vi "todos los modulos.vi"() -> ()   [LabVIEW 2010]
uses:
  <vilib>/sound2/lvsound2.llb/Sound Data Format.ctl
  <vilib>/addons/PixeLINK/Low Level Functions/CAMERA_FEATURES.llb/TDPU-CameraFeatures-PixelFormat.ctl
  <vilib>/sound2/lvsound2.llb/Sound Output Task ID.ctl
  <vilib>/vision/Image Controls.llb/IMAQ Image.ctl
panel:
  in  "Tab Control":enum32{"DAQ", "Sound", "Camara"}(tab)
  out "Waveform DAQ":waveform(dbl)(graph)
  in  "Calibracion DAQ":T1
  in  "DAQ Controls":T2={"Minimum Value"=-10.0, "Maximum Value"=10.0, "Physical Channel"="Dev1/ao0", "DAQ Fs (S/s)"=10000.0} {"Minimum Value" min=-10.0 max=0.0; "Maximum Value" min=0.0 max=10.0}
  in  "tiempo (ms)":dbl
  in  "DAQ?":bool
  in  "Sound Controls":T4={"device ID"=0, "sound format"={"sample rate (S/s)"=44000.0, "number of channels"=2, "bits per sample"=16}, "time (ms)"=200.0}
  in  "Sound?":bool
  in  "Frecuencia":dbl
  out "Waveform Sound":waveform(dbl)(graph)
  in  "Selector":u16(ring) items=["776002034"]
  in  "Streeam?":bool
  in  "Camera Parameters":T6 {"Pixel Format" items=["PIXEL_FORMAT_MONO8", "PIXEL_FORMAT_MONO16", "PIXEL_FORMAT_YUV422", "PIXEL_FORMAT_BAYER8_GRBG", "PIXEL_FORMAT_BAYER16_GRBG", "PIXEL_FORMAT_RGB24", "PIXEL_FORMAT_RGB48", "PIXEL_FORMAT_BAYER8_RGGB", "PIXEL_FORMAT_BAYER8_GBRG ", "PIXEL_FORMAT_BAYER8_BGGR ", "PIXEL_FORMAT_BAYER16_RGGB ", "PIXEL_FORMAT_BAYER16_GBRG", "PIXEL_FORMAT_BAYER16_BGGR", "PIXEL_FORMAT_RGB32"]}
  out "Camara Funciona?":bool
  out "Contraste":dbl
  out "Image":T7(plugin-control)
  in  "stop":bool
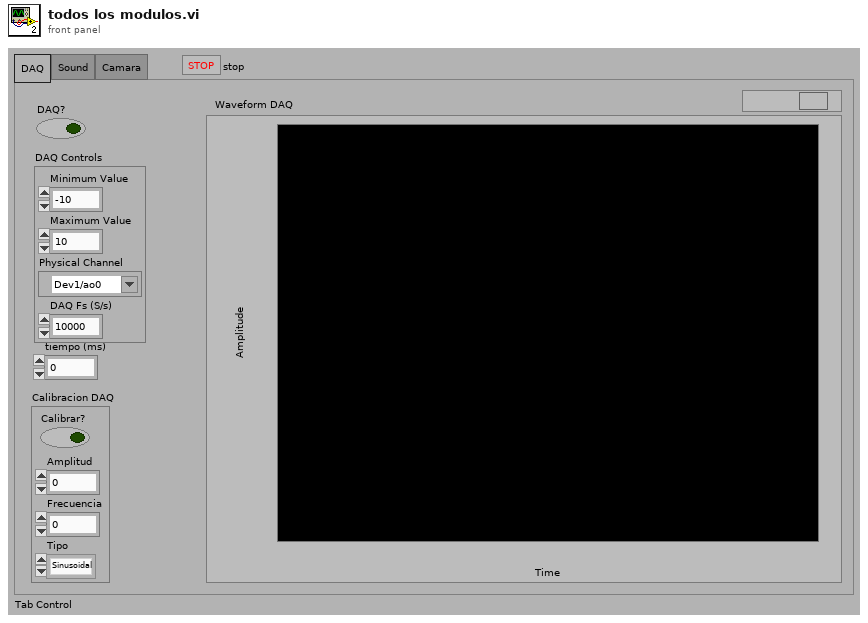
[diagram p1: front panel]
types:
  T1 = cluster{"Calibrar?":bool, "Amplitud":dbl, "Frecuencia":dbl, "Tipo":enum16{"Sinusoidal", "Triangular", "Cuadrada"}}
  T2 = cluster{"Minimum Value":dbl, "Maximum Value":dbl, "Physical Channel":tag, "DAQ Fs (S/s)":dbl}
  T3 = typedef "Sound Data Format.ctl" = cluster{"sample rate (S/s)":dbl, "number of channels":i32, "bits per sample":i32}
  T4 = cluster{"device ID":u32, "sound format":T3, "time (ms)":dbl}
  T5 = typedef "TDPU-CameraFeatures-PixelFormat.ctl" = u16
  T6 = cluster{"Exposure Time (ms)":u32, "Gain (dB)":dbl, "Saturation (%)":dbl, "Brightness (%)":dbl, "Color Temperature":dbl, "ROI":cluster{"Top":i32, "Left":i32, "Width":i32, "Height":i32}, "White Balance Gain (dB)":cluster{"Red":dbl, "Green":dbl, "Blue":dbl}, "Gamma":dbl, "Pixel Format":T5}
  T7 = typedef "IMAQ Image.ctl" = refnum<image>
  T8 = cluster{"hCamera":u32, "Error":errorcluster, "uSerialNumber OUT":u32}
  T9 = typedef "Sound Output Task ID.ctl" = u32
  T10 = cluster{"task ID":T9, "error":errorcluster, "sound format":T3}
  T11 = cluster{"DAQ Fs (S/s)":dbl, "task":refnum<k21>, "error":errorcluster, "Min Value":dbl, "Max Value":dbl}
  T12 = cluster{"DAQ Limits":cluster{"max":dbl, "min":dbl}, "Control Limits":cluster{"max":dbl, "min":dbl}}
  T13 = cluster{"hCamera":u32, "Error":errorcluster, "uSerialNumber":u32}
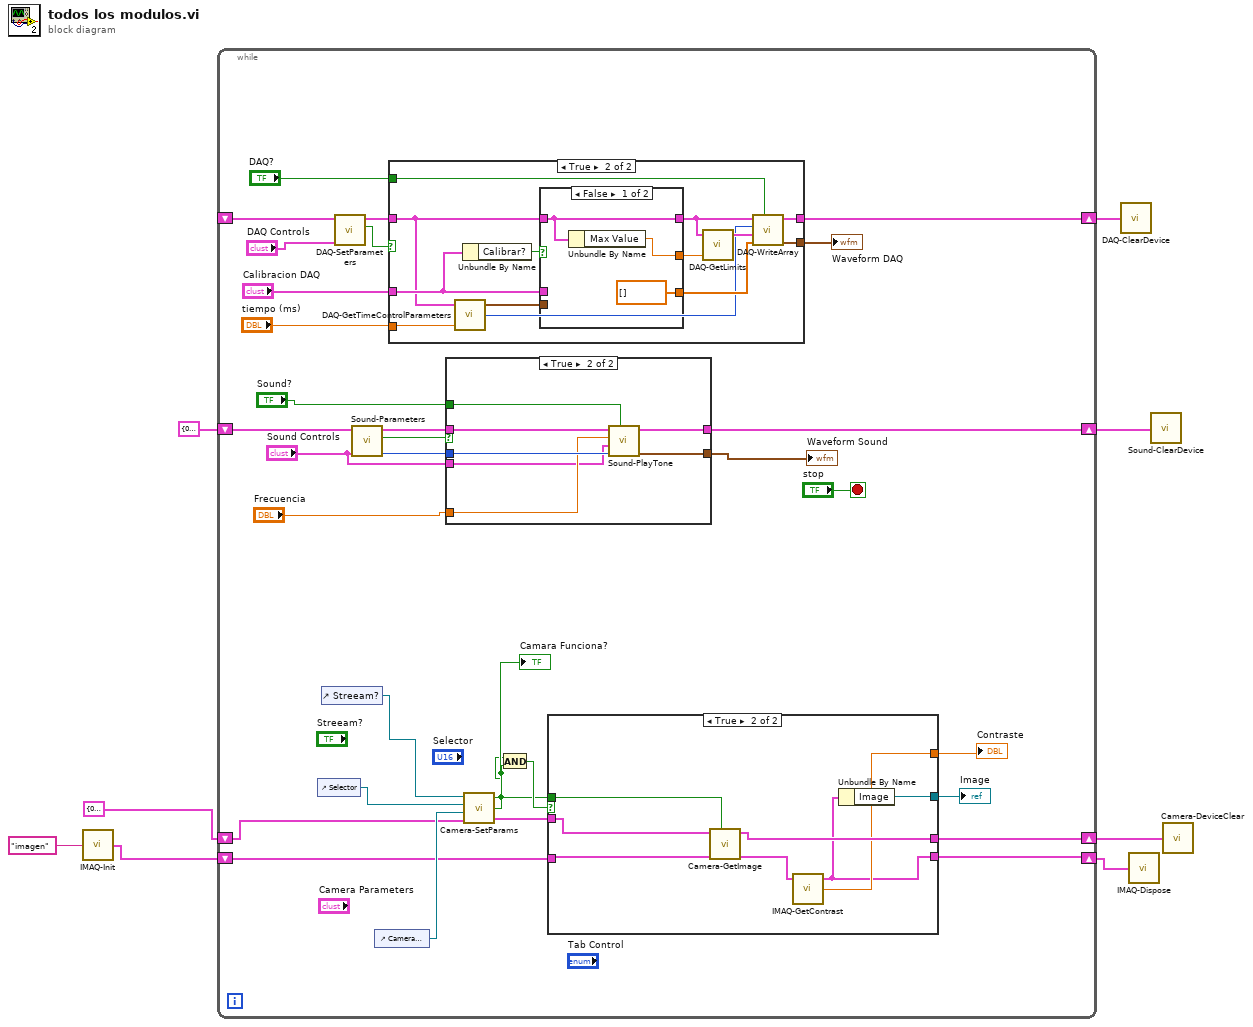
[diagram p0: block diagram]
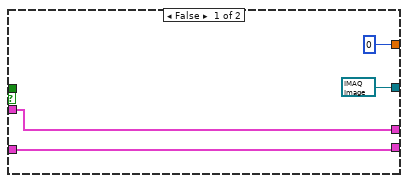
[diagram p2: hidden frame]
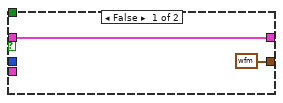
[diagram p3: hidden frame]
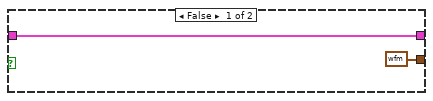
[diagram p4: hidden frame]
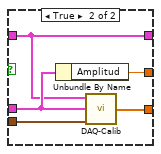
[diagram p5: hidden frame]
diagram:
  n1 = call "IMAQ-Init.vi"("Image Name"="imagen") -> ("Image Device IN"=w4:cluster{"Image":T7, "errorImage":errorcluster})
  n2 = while {
    shift-right: [w32] -> w6
    shift-left: _ -> [w33]
    shift-right: [w28] -> w7
    shift-left: T10 {"task ID"=0, "error"={"status"=TRUE, "code"=0, "source"=""}, "sound format"={"sample rate (S/s)"=0.0, "number of channels"=0, "bits per sample"=0}} ("Sound Device OUT") -> [w27]
    shift-right: [w13] -> w1
    shift-left: w4 -> [w17]
    shift-right: [w16] -> w2
    shift-left: T8 {"hCamera"=0, "Error"={"status"=FALSE, "code"=0, "source"=""}, "uSerialNumber OUT"=0} ("Camera Device  IN") -> [w15]
    stop <- "stop" stop-if-true
    n3 = control-ref of="Selector"() -> (w21:refnum<vi>)
    n4 = control-ref of="Streeam?"() -> (w19:refnum<vi>)
    n5 = call "DAQ-SetParameters.vi"("DAQ Controls"="DAQ Controls", "DAQ Device IN"=w33) -> ("En Funcionamiento?"=w26:bool, "DAQ Device OUT"=w38:T11)  [unwired: 4 in]
    n6 = call "Sound-Parameters.vi"("Sound Controls"="Sound Controls", "Sound Device IN"=w27) -> ("#samples"=w29:u32, "En funcionamiento?"=w25:bool, "Sound Device OUT"=w30:T10)  [unwired: 3 in]
    n7 = control-ref of="Camera Parameters"() -> (w20:refnum<vi>)
    n8 = case shown="True" w26 {
      tunnel: "DAQ?" -> [_ w74]
      tunnel: w38 -> [w63 w65]
      tunnel: [waveform(dbl) {"t0"=timestamp(0 s since 1904-01-01), "dt"=1.0, "Y"=[]} ("Waveform Graph") w71] -> w37
      tunnel: "Calibracion DAQ" -> [_ w67]
      tunnel: "tiempo (ms)" -> [_ w69]
      tunnel: [w63 w68] -> w32
      frame False {
      }
      frame True {
        n9 = call "DAQ-GetTimeControlParameters.vi"("tiempo (ms)"=w69, "DAQ Device IN"=w65) -> ("#samples"=w72:u32, "Time Control Parameters"=w73:cluster{"# samples":u32, "tiempos (ms)":dbl})  [unwired: 2 in]
        n10 = Unbundle By Name(w67) -> ("Calibrar?"=w66:bool)
        n11 = case shown="False" w66 {
          tunnel: [dbl[] [] ("Calibration OUT") w84] -> w76
          tunnel: w73 -> [_ w83]
          tunnel: w65 -> [w77 w80]
          tunnel: w67 -> [_ w82]
          tunnel: [w78 w81] -> w70
          tunnel: [w77 w80] -> w64
          frame False {
            n12 = Unbundle By Name(w77) -> ("Max Value"=w78:dbl)
          }
          frame True {
            n13 = Unbundle By Name(w82) -> ("Amplitud"=w81:dbl)
            n14 = call "DAQ-Calib.vi"("Time Control Parameters"=w83, "Calibracion DAQ"=w82, "DAQ Device IN"=w80) -> ("Calibration OUT"=w84:dbl[])  [unwired: 1 in]
          }
        }
        n15 = call "DAQ-GetLimits.vi"("Amplitud"=w70, "DAQ Device IN"=w64) -> ("Limites"=w75:T12)  [unwired: 3 in]
        n16 = call "DAQ-WriteArray.vi"("DAQ?"=w74, "Control Array"=w76, "Limites"=w75, "#samples"=w72, "DAQ Device IN"=w64) -> ("Waveform Graph"=w71:waveform(dbl), "DAQ Device OUT"=w68:T11)  [unwired: 2 in]
      }
    }
    "Waveform DAQ" <- w37
    n17 = case shown="True" w25 {
      tunnel: [waveform(dbl) {"t0"=timestamp(0 s since 1904-01-01), "dt"=1.0, "Y"=[]} ("Waveform") w61] -> w31
      tunnel: w30 -> [w54 w60]
      tunnel: w29 -> [_ w59]
      tunnel: [w54 w58] -> w28
      tunnel: "Sound?" -> [_ w57]
      tunnel: "Frecuencia" -> [_ w56]
      tunnel: "Sound Controls" -> [_ w55]
      frame False {
      }
      frame True {
        n18 = call "Sound-PlayTone.vi"("sound?"=w57, "# samples"=w59, "Sound Controls"=w55, "Frecuencia"=w56, "Sound Device IN"=w60) -> ("Waveform"=w61:waveform(dbl), "Sound Device OUT"=w58:T10)  [unwired: 3 in]
      }
    }
    "Waveform Sound" <- w31
    n19 = call "Camera-SetParams.vi"("Camera Device  IN"=w15, "Camera Parameters"=w20, "Selector"=w21, "Stream?"=w19) -> ("Camera Device OUT"=w18:T13, "Funciona?"=w11:bool, "Stream? OUT"=w10:bool)
    "Camara Funciona?" <- w11
    n20 = And(x=w10, y=w11) -> (x .and. y?=w12:bool)
    n21 = case shown="True" w12 {
      tunnel: w18 -> [w44 w51]
      tunnel: w10 -> [_ w52]
      tunnel: w17 -> [w43 w50]
      tunnel: [w44 w49] -> w16
      tunnel: [T7 refnum ("Image") w48] -> w14
      tunnel: [w43 w45] -> w13
      tunnel: [u32 0 ("Numeric") w47] -> w9
      frame False {
      }
      frame True {
        n22 = call "Camera-GetImage.vi"("Streeam"=w52, "Image Device IN"=w50, "Camera Device IN"=w51) -> ("Image Device OUT"=w46:cluster{"Image":T7, "errorImage":errorcluster}, "Camera Device OUT"=w49:T13)  [unwired: 4 in]
        n23 = call "IMAQ-GetContrast.vi"("Image Device IN"=w46) -> ("Contraste"=w47:dbl, "Image Device OUT"=w45:cluster{"Image":T7, "errorImage":errorcluster})  [unwired: 3 in]
        n24 = Unbundle By Name(w45) -> ("Image"=w48:T7)
      }
    }
    "Image" <- w14
    "Contraste" <- w9
  }
  n25 = call "DAQ-ClearDevice.vi"("DAQ Device IN"=w6) -> ()
  n26 = call "IMAQ-Dispose.vi"("Image Device IN"=w1) -> ()
  n27 = call "Sound-ClearDevice.vi"("Sound Device OUT"=w7) -> ()
  n28 = call "Camera-DeviceClear.vi"("Camera Device OUT"=w2) -> ()
